vi "Alternate Mark Inversion.vi"(4 "Phase In":dbl format="%.2f", 5 "Sampling Frequency":dbl=100000000.0 format="%.2e", 6 "Frequency":dbl=1544000.0 format="%.2e", 7 "Amplitude":dbl format="%.2f", 8 "Line Code":string) -> (0 "Phase Out":dbl format="%.2f", 1 "Samples Generated":i32, 2 "Signal":dbl[](array[numeric]) format="%.2f", 3 "Time Axis":dbl[](array[numeric]) format="%.2f")   [LabVIEW 2012]
doc: "Input phase of the signal"
panel:
  out "Waveform Graph":dbl[](graph)
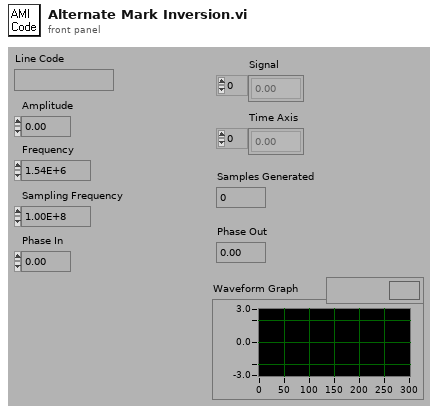
[diagram p1: front panel]
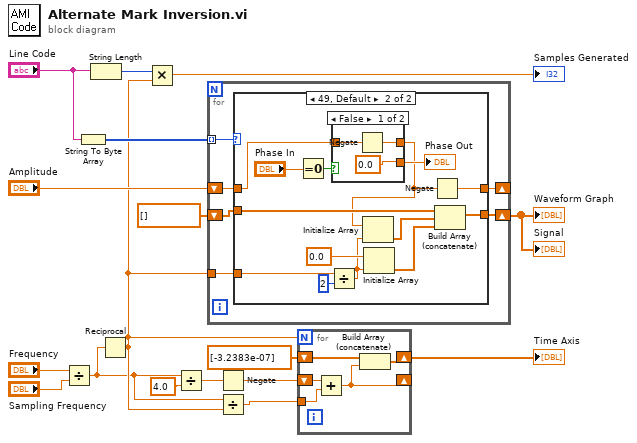
[diagram p0: block diagram]
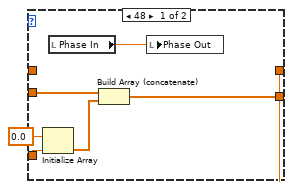
[diagram p2: hidden frame]
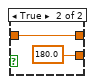
[diagram p3: hidden frame]
diagram:
  n1 = Divide(x="Frequency", y="Sampling Frequency") -> (x/y=w1:dbl)
  n2 = String To Byte Array(string="Line Code") -> (unsigned byte array=w14:u8[])
  n3 = String Length(string="Line Code") -> (length=w17:i32)
  n4 = Reciprocal(x=w1) -> (1/x=w5:dbl)
  n5 = Multiply(x=w17, y=w5) -> (x*y=→"Samples Generated":dbl)
  n6 = Divide(x=w1, y=4.0) -> (x/y=w11:dbl)
  n7 = for {
    tunnel: w14 -> [w23] mode=indexing
    tunnel: w5 -> [w22]
    shift-right: [w21] -> w4
    shift-left: dbl[] [] -> [w20]
    shift-right: [w19] -> _
    shift-left: "Amplitude" -> [w18]
    n8 = case shown="49, Default" w23 {
      tunnel: w22 -> [w29 w43]
      tunnel: [w27 w39] -> w21
      tunnel: w20 -> [w26 w40]
      tunnel: [w25 w36] -> w19
      tunnel: w18 -> [w25 w32]
      frame 48 {
        n9 = Initialize Array(0.0 ("Element Data"), w29) -> (w28:dbl[])
        n10 = local read "Phase In"() -> (w24:dbl)
        n11 = Build Array (concatenate)(w26, w28) -> (w27:dbl[])
        n12 = local write "Phase Out"(w24) -> ()
      }
      frame 49, Default {
        n13 = Equal To 0?(x="Phase In") -> (x = 0?=w34:bool)
        n14 = Divide(x=w43, y=2) -> (x/y=w41:dbl)
        n15 = case shown="False" w34 {
          tunnel: [0.0 180.0] -> w33
          tunnel: w32 -> [w47 w48]
          tunnel: [w46 w48] -> w31
          frame False {
            n16 = Negate(x=w47) -> (-x=w46:dbl)
          }
          frame True {
          }
        }
        "Phase Out" <- w33
        n17 = Initialize Array(w31, w41) -> (w38:dbl[])
        n18 = Initialize Array(0.0 ("Element Data"), w41) -> (w37:dbl[])
        n19 = Negate(x=w31) -> (-x=w36:dbl)
        n20 = Build Array (concatenate)(w40, w38, w37) -> (w39:dbl[])
      }
    }
  }
  "Signal" <- w4
  "Waveform Graph" <- w4
  n21 = Negate(x=w11) -> (-x=w7:dbl)
  n22 = Divide(x=w1, y=w5) -> (x/y=w10:dbl)
  n23 = for {
    N: w5 -> [_]
    shift-right: [w52] -> _
    shift-left: w7 -> [w54]
    tunnel: w10 -> [w53]
    shift-right: [w50] -> w9
    shift-left: dbl[] [-3.2383e-07] -> [w51]
    n24 = Add(x=w54, y=w53) -> (x+y=w52:dbl)
    n25 = Build Array (concatenate)(w51, w52) -> (w50:dbl[])
  }
  "Time Axis" <- w9
